vi "ReportPart_A131258.vi"(6 "试验项目":enum32{"压装"}(ring), 8 "error in":errorcluster, 9 "索引":i32, 10 "合格":T1, 11 "report in":refnum<class "NI_report.lvclass">) -> (0 "error out 2":errorcluster caption="error out", 3 "report out":refnum<class "NI_report.lvclass">)   [LabVIEW 2020]
uses:
  <vilib>/Utility/NIReport.llb/NI_report.lvclass
  OK.ctl
  <vilib>/Utility/NIReport.llb/image depth.ctl
  <vilib>/addons/_office/_exclsub.llb/font.ctl
  Global_Variable/A131258.vi
  <vilib>/Utility/NIReport.llb/Append Report Text (str wrap).vi
  Global_Variable/Global.vi
  <vilib>/addons/_office/word.llb/Word Easy Table (str).vi
  <vilib>/Utility/NIReport.llb/NI_ReportGenerationCore.lvlib
  <vilib>/Utility/NIReport.llb/Word/NI_Word.lvclass
  <vilib>/addons/_office/NI_ReportGenerationToolkit.lvlib
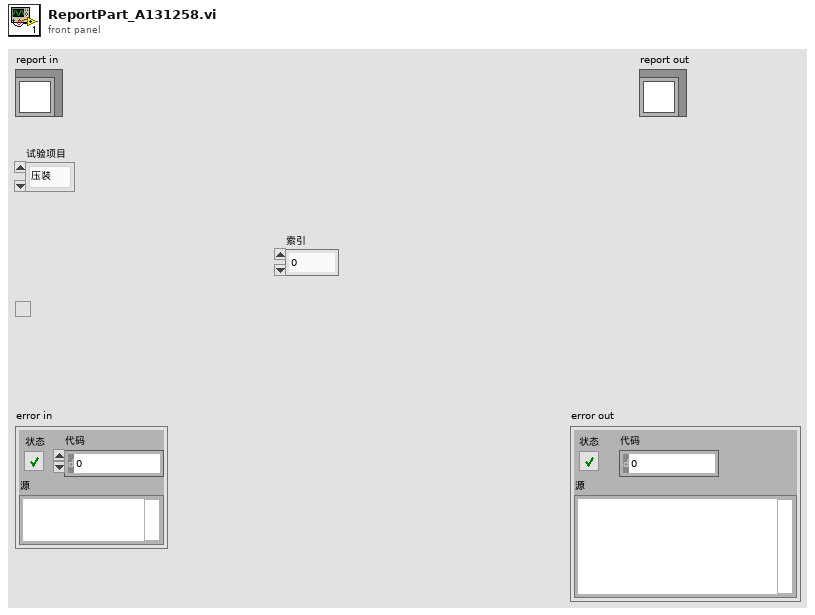
[diagram p1: front panel]
types:
  T1 = typedef "OK.ctl" = bool
  T2 = cluster{"Charset (-1)":i16, "Weight (-1)":i16, "Name":string, "Size":string}
  T3 = cluster{"Italic":enum16{"Italic Unchanged", "Italic On", "Italic Off"}, "Strike Through":enum16{"Strike Through Unchanged", "Strike Through On", "Strike Through Off"}, "Underline":enum16{"Underline Unchanged", "Underline On", "Underline Off"}, "Bold":enum16{"Bold Unchanged", "Bold On", "Bold Off"}}
  T4 = typedef "NI_ReportGenerationToolkit.lvlib/font.ctl" = cluster{"font name":string, "font size":dbl, "bold":u16, "italic":u16, "underline":u16, "strike through":u16, "font color":u32}
  T5 = typedef "NI_ReportGenerationCore.lvlib/image depth.ctl" = u16
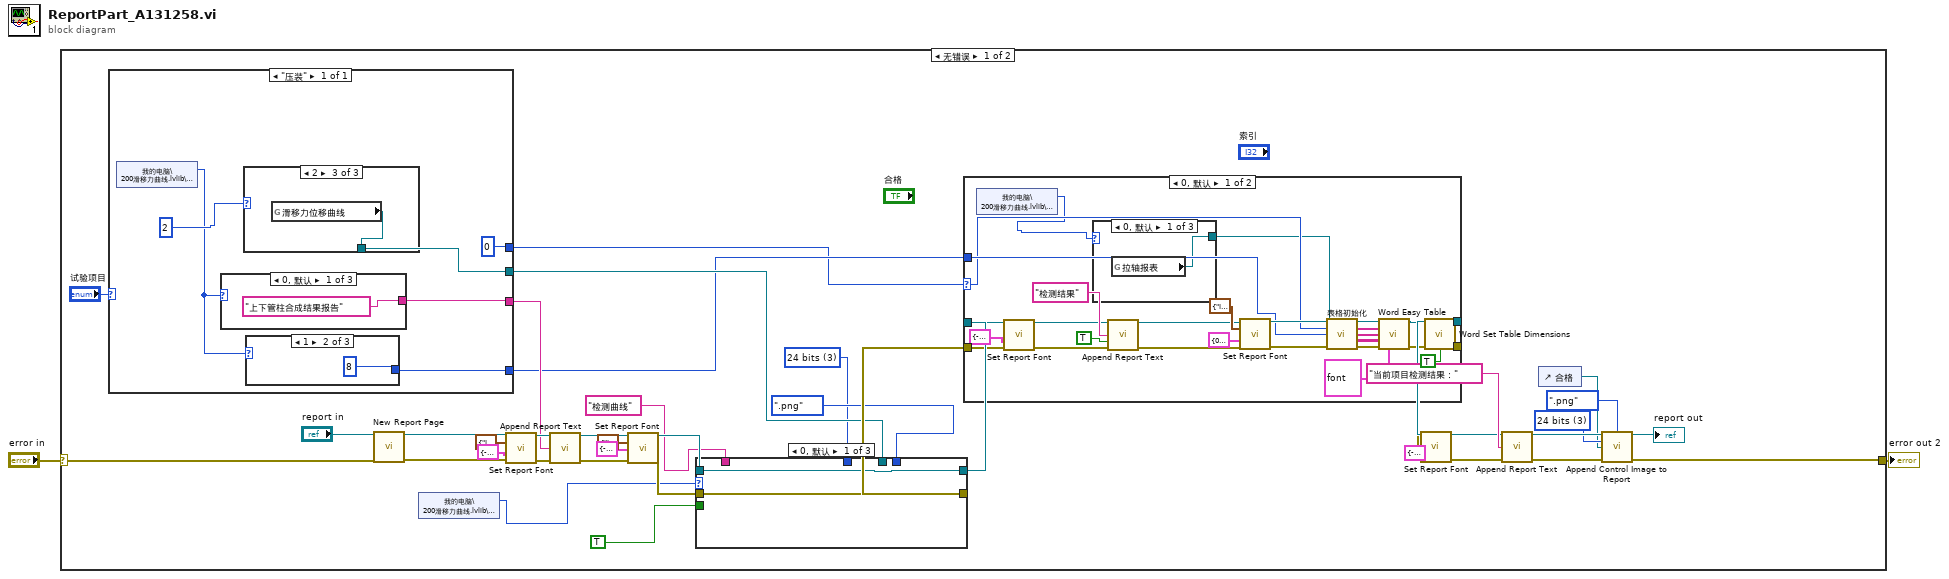
[diagram p0: block diagram]
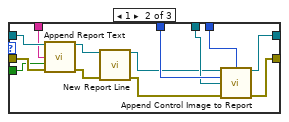
[diagram p2: hidden frame]
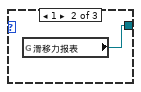
[diagram p4: hidden frame]
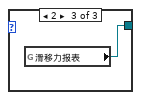
[diagram p5: hidden frame]
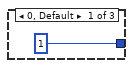
[diagram p7: hidden frame]
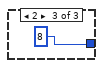
[diagram p8: hidden frame]
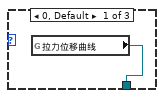
[diagram p9: hidden frame]
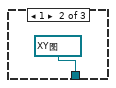
[diagram p10: hidden frame]
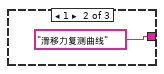
[diagram p11: hidden frame]
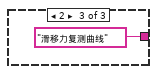
[diagram p12: hidden frame]
diagram:
  n1 = case shown="无错误" "error in" {
    selector: "error in" -> [w25 w106]
    tunnel: [w19 w106] -> w1
    frame No Error {
      w6 = T5 3 items=["B&W", "4 bits", "8 bits", "24 bits"] ("image depth")
      w17 = T5 3 items=["B&W", "4 bits", "8 bits", "24 bits"] ("image depth")
      n2 = case shown="\"压装\"" "试验项目" {
        tunnel: [w95] -> w9
        tunnel: [w94] -> w36
        tunnel: [w93] -> w8
        tunnel: [0 ("长度")] -> w4
        frame "压装" {
          n3 = shared-variable "我的电脑\\200滑移力曲线.lvlib\\备用_5"() -> (w91:u16)  [unwired: 1 in, 1 out]
          n4 = case shown="0, 默认" w91 {
            tunnel: ["上下管柱合成结果报告" ("text") "滑移力复测曲线" ("text") "滑移力复测曲线" ("text")] -> w94
            frame 0, Default {
            }
            frame 1 {
            }
            frame 2 {
            }
          }
          n5 = case shown="2" 2 {
            tunnel: [w100 refnum<vi> refnum ("拉力位移曲线") w102] -> w95
            frame 0, Default {
              n6 = global read "A131258.vi" "拉力位移曲线"() -> (w100:refnum<vi>)
            }
            frame 1 {
            }
            frame 2 {
              n7 = global read "A131258.vi" "滑移力位移曲线"() -> (w102:refnum<vi>)
            }
          }
          n8 = case shown="1" w91 {
            tunnel: [1 8 8 ("长度")] -> w93
            frame 0, Default {
            }
            frame 1 {
            }
            frame 2 {
            }
          }
        }
      }
      n9 = call-dynamic "New Report Page.vi"("report in"="report in", "error in (no error)"=w25) -> ("report out"=w23:refnum<class "NI_report.lvclass">, "error out"=w24:errorcluster)  [unwired: 12 in]
      n10 = shared-variable "我的电脑\\200滑移力曲线.lvlib\\备用_5"() -> (w3:u16)  [unwired: 1 in, 1 out]
      n11 = call-dynamic "Set Report Font.vi"("report in"=w23, "text options"=T3 {"Italic"=enum."Italic Unchanged", "Strike Through"=enum."Strike Through Unchanged", "Underline"=enum."Underline Unchanged", "Bold"=enum."Bold On"}, "font settings"=T2 {"Charset (-1)"=-1, "Weight (-1)"=-1, "Name"="楷体", "Size"="16 "}, "error in (no error)"=w24) -> ("report out"=w41:refnum<class "NI_report.lvclass">, "error out"=w40:errorcluster)  [unwired: 9 in, 1 out]
      n12 = call-poly <vilib>:"Append Report Text.vi"("report in"=w41, "text"=w36, "error in (no error)"=w40) -> ("report out"=w33:refnum<class "NI_report.lvclass">, "error out"=w32:errorcluster)  [unwired: 9 in, 2 out]
      n13 = call-dynamic "Set Report Font.vi"("report in"=w33, "text options"=T3 {"Italic"=enum."Italic Unchanged", "Strike Through"=enum."Strike Through Unchanged", "Underline"=enum."Underline Unchanged", "Bold"=enum."Bold Off"}, "font settings"=T2 {"Charset (-1)"=-1, "Weight (-1)"=-1, "Name"="宋体", "Size"="12 "}, "error in (no error)"=w32) -> ("report out"=w29:refnum<class "NI_report.lvclass">, "error out"=w28:errorcluster)  [unwired: 9 in, 1 out]
      n14 = case shown="0, 默认" w3 {
        tunnel: [w43 w45 w58] -> w38
        tunnel: [w42 w44 w57] -> w37
        tunnel: w29 -> [w43 w53 w58]
        tunnel: w28 -> [w42 w51 w57]
        tunnel: TRUE ("append on new line? (F)") -> [_ w50 _]
        tunnel: w9 -> [_ w54 _]
        tunnel: enum16{".jpg", ".png"}.".png" ("image file type (.jpg)") -> [_ w56 _]
        tunnel: w6 -> [_ w55 _]
        tunnel: "检测曲线" ("text") -> [_ w52 _]
        frame 0, Default {
        }
        frame 1 {
          n15 = call-poly <vilib>:"Append Report Text.vi"("report in"=w53, "text"=w52, "append on new line? (F)"=w50, "error in (no error)"=w51) -> ("report out"=w49:refnum<class "NI_report.lvclass">, "error out"=w48:errorcluster)  [unwired: 8 in, 2 out]
          n16 = call-dynamic "New Report Line.vi"("report in"=w49, "error in (no error)"=w48) -> ("report out"=w47:refnum<class "NI_report.lvclass">, "error out"=w46:errorcluster)  [unwired: 12 in]
          n17 = call-dynamic "Append Control Image to Report.vi"("report in"=w47, "image file type (.jpg)"=w56, "image depth"=w55, "ctrl reference"=w54, "error in (no error)"=w46) -> ("report out"=w45:refnum<class "NI_report.lvclass">, "error out"=w44:errorcluster)  [unwired: 7 in, 2 out]
        }
        frame 2 {
        }
      }
      n18 = case shown="0, 默认" w4 {
        selector: w4 -> [w61 _]
        tunnel: w38 -> [w81 w90]
        tunnel: w37 -> [w79 w89]
        tunnel: [w66 w90] -> w11
        tunnel: [w65 w89] -> w10
        tunnel: w8 -> [w62 _]
        frame 0, Default {
          n19 = shared-variable "我的电脑\\200滑移力曲线.lvlib\\备用_5"() -> (w59:u16)  [unwired: 1 in, 1 out]
          n20 = call-dynamic "Set Report Font.vi"("report in"=w81, "font settings"=T2 {"Charset (-1)"=-1, "Weight (-1)"=-1, "Name"="宋体", "Size"="12 "}, "error in (no error)"=w79) -> ("report out"=w82:refnum<class "NI_report.lvclass">, "error out"=w80:errorcluster)  [unwired: 10 in, 1 out]
          n21 = case shown="0, 默认" w59 {
            tunnel: [w86 w87 w88] -> w60
            frame 0, Default {
              n22 = global read "Global.vi" "拉轴报表"() -> (w86:refnum<vi>)
            }
            frame 1 {
              n23 = global read "Global.vi" "滑移力报表"() -> (w87:refnum<vi>)
            }
            frame 2 {
              n24 = global read "Global.vi" "滑移力报表"() -> (w88:refnum<vi>)
            }
          }
          n25 = call-poly <vilib>:"Append Report Text.vi"("report in"=w82, "text"="检测结果", "append on new line? (F)"=TRUE, "error in (no error)"=w80) -> ("report out"=w64:refnum<class "NI_report.lvclass">, "error out"=w63:errorcluster)  [unwired: 8 in, 2 out]
          n26 = call-dynamic "Set Report Font.vi"("report in"=w64, "text options"=T3 {"Italic"=enum."Italic Unchanged", "Strike Through"=enum."Strike Through Unchanged", "Underline"=enum."Underline Unchanged", "Bold"=enum."Bold Unchanged"}, "font settings"=T2 {"Charset (-1)"=0, "Weight (-1)"=-1, "Name"="微软雅黑", "Size"="12 "}, "error in (no error)"=w63) -> ("report out"=w68:refnum<class "NI_report.lvclass">, "error out"=w67:errorcluster)  [unwired: 9 in, 1 out]
          n27 = call "表格初始化.vi"("表格引用"=w60, "索引"=w61, "长度"=w62, "错误输入（无错误）"=w67) -> ("行首字符串[]"=w70:string[], "列首字符串[]"=w69:string[], "文本数据"=w72:string[][], "错误输出"=w75:errorcluster)  [unwired: 7 in, 1 out]
          n28 = call-poly <vilib>:"Word Easy Table.vi"("report in"=w68, "row headers"=w70, "column headers"=w69, "data"=w72, "error in (no error)"=w75, "font"=T4 {"font name"="宋体", "font size"=12.0, "bold"=2, "italic"=2, "underline"=2, "strike through"=2, "font color"=16777216}) -> ("report out"=w73:refnum<class "NI_report.lvclass">, "error out"=w74:errorcluster)  [unwired: 7 in, 1 out]
          n29 = call <vilib>:"Word Set Table Dimensions.vi"("report in"=w73, "error in (no error)"=w74, "fit to page width? (F)"=TRUE) -> ("report out"=w66:refnum<class "NI_report.lvclass">, "error out"=w65:errorcluster)  [unwired: 11 in]
        }
        frame -1 {
        }
      }
      n30 = call-dynamic "Set Report Font.vi"("report in"=w11, "font settings"=T2 {"Charset (-1)"=-1, "Weight (-1)"=-1, "Name"="宋体", "Size"="16 "}, "error in (no error)"=w10) -> ("report out"=w14:refnum<class "NI_report.lvclass">, "error out"=w15:errorcluster)  [unwired: 10 in, 1 out]
      n31 = call-poly <vilib>:"Append Report Text.vi"("report in"=w14, "text"="当前项目检测结果：", "error in (no error)"=w15) -> ("report out"=w22:refnum<class "NI_report.lvclass">, "error out"=w20:errorcluster)  [unwired: 9 in, 2 out]
      n32 = control-ref of="合格"() -> (w16:refnum<vi>)
      n33 = call-dynamic "Append Control Image to Report.vi"("report in"=w22, "image file type (.jpg)"=enum16{".jpg", ".png"}.".png", "image depth"=w17, "ctrl reference"=w16, "error in (no error)"=w20) -> ("report out"=→"report out":refnum<class "NI_report.lvclass">, "error out"=w19:errorcluster)  [unwired: 7 in, 2 out]
    }
    frame Error {
    }
  }
  "error out 2" <- w1
